vi "Test.vi"   [LabVIEW 2017]
doc: "Builds all of the build specifications defined in this project."
uses:
  tests/Tests.lvlib
  <vilib>/addons/_JKI Toolkits/Caraya/classes/Test/Test.lvclass
panel:
  # "Overview: Runs all of tests this project\nRequirements: LabVIEW\nInstructions: Run this VI.\n\nThis VI runs all of the integration and unit tests."
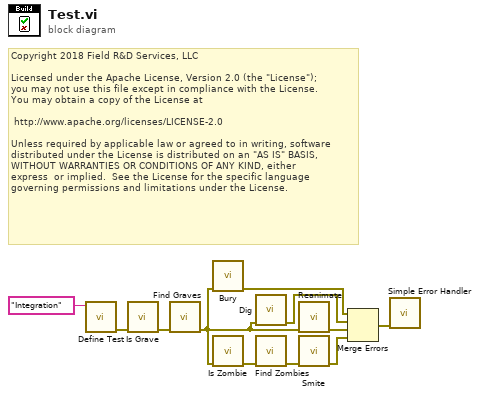
[diagram p0: block diagram]
diagram:
  # "Copyright 2018 Field R&D Services, LLC\n\nLicensed under the Apache License, Version 2.0 (the \"License\");\nyou may not use this file except in compliance with the License.\nYou may obtain a copy of the License at\n\n\thttp://www.apache.org/licenses/LICENSE-2.0\n\nUnless required by applicable law or agreed to in writing, software\ndistributed under the License is distributed on an \"AS IS\" BASIS,\nWITHOUT WARRANTIES OR CONDITIONS OF ANY KIND, either \nexpress  or implied.  See the License for the specific language \ngoverning permissions and limitations under the License."
  n1 = call <vilib>:"Define Test.vi"("Label (VI Title)"="Integration") -> ("error out"=w4:errorcluster)  [unwired: 10 in]
  n2 = call "Is Grave.vi"("Error In"=w4) -> ("Error Out"=w3:errorcluster)  [unwired: 10 in]
  n3 = call "Find Graves.vi"("Error In"=w3) -> ("Error Out"=w1:errorcluster)  [unwired: 10 in]
  n4 = call "Bury.vi"("Error In"=w1) -> ("Error Out"=w11:errorcluster)  [unwired: 10 in]
  n5 = call "Is Zombie.vi"("Error In"=w1) -> ("Error Out"=w2:errorcluster)  [unwired: 10 in]
  n6 = call "Dig.vi"("Error In"=w1) -> ("Error Out"=w10:errorcluster)  [unwired: 10 in]
  n7 = call "Find Zombies.vi"("Error In"=w2) -> ("Error Out"=w5:errorcluster)  [unwired: 10 in]
  n8 = call "Reanimate.vi"("Error In"=w1) -> ("Error Out"=w9:errorcluster)  [unwired: 10 in]
  n9 = call "Smite.vi"("Error In"=w5) -> ("Error Out"=w8:errorcluster)  [unwired: 10 in]
  n10 = Merge Errors(w11, w10, w9, w8) -> (w7:errorcluster)
  n11 = call <vilib>:"Simple Error Handler.vi"("error in (no error)"=w7) -> ()  [unwired: 4 in, 5 out]
